vi "XY Graph Delete Plot.vi"(8 "Error In":errorcluster, 9 "Plot Index":i32, 11 "XYGraph Ref":T1) -> (0 "Error Out":errorcluster, 2 "Plot Name":string, 3 "XYGraph Ref":T1, 5 "Graph Caption (or Label)":string)   [LabVIEW 2019, in "XY Graph Add-Ons.lvlib"]
uses:
  XY Graph Add-Ons.lvlib
  XY Graph Refnum.ctl
  Plot Update Steps.ctl
  XY Graph Plot Properties.ctl
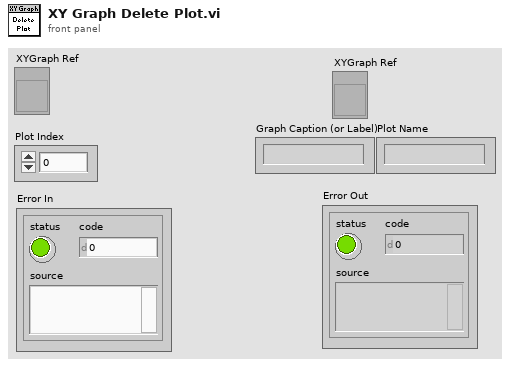
[diagram p1: front panel]
types:
  T1 = typedef "XY Graph Add-Ons.lvlib/XY Graph Refnum.ctl" = refnum<vi>
  T2 = typedef "Plot Update Steps.ctl" = enum16{"Update Plot Styles", "Update Annotation List", "Update Cursor List", "Update Plots", "Quit"}
  T3 = typedef "XY Graph Plot Properties.ctl" = cluster{"Plot Index":i32, "Plot.Bar Plot Style":u8, "Plot.DigitalLineStyle":u8, "Plot.TransitionLocation":u8, "Plot.Transition Type":u8, "Plot.Fill To":i16, "Plot.Fill/Pt. Color":u32, "Plot.Label Format":u8, "Plot.Line Style":u8, "Plot.Line Width":u8, "Plot.Plot Color":u32, "Plot.Plot Interpolation":u8, "Plot.Plot Name":string, "Plot.Point Style":u8, "Plot.Visible?":bool, "Plot.XScaleIdx":u32, "Plot.YScaleIdx":u32, "Plot.Anti-aliased":bool}
  T4 = typedef "LVAnnotationListTypeDef.ctl" = cluster{"Name":string, "Color":u32, "Style":u8, "Point Style":u8, "Name Visible":bool, "Allow Drag":bool, "Annotation Mode":u32, "Plot":i32, "Index":i32, "Position":cluster{"X":dbl, "Y":dbl}, "X Scale":u32, "Y Scale":u32, "Show Arrow":bool, "Lock Name":bool, "Plot Area":i32, "Label Offset":cluster{"X":dbl, "Y":dbl}}[]
  T5 = typedef "LVCursorListTypeDef.ctl" = cluster{"Name":string, "Color":u32, "Style":u8, "Point Style":u8, "Name Visible":bool, "Allow Drag":bool, "Cursor Mode":u32, "Plot":i32, "Index":i32, "Position":cluster{"X":dbl, "Y":dbl}, "X Scale":u32, "Y Scale":u32, "Watch Plots":i32[], "Watch All Plots":bool, "Plot Area":i32, "Label Offset":cluster{"X":dbl, "Y":dbl}}[]
  T6 = cluster{"Name":string, "Color":u32, "Style":u8, "Point Style":u8, "Name Visible":bool, "Allow Drag":bool, "Annotation Mode":u32, "Plot":i32, "Index":i32, "Position":cluster{"X":dbl, "Y":dbl}, "X Scale":u32, "Y Scale":u32, "Show Arrow":bool, "Lock Name":bool, "Plot Area":i32, "Label Offset":cluster{"X":dbl, "Y":dbl}}
  T7 = cluster{"Name":string, "Color":u32, "Style":u8, "Point Style":u8, "Name Visible":bool, "Allow Drag":bool, "Cursor Mode":u32, "Plot":i32, "Index":i32, "Position":cluster{"X":dbl, "Y":dbl}, "X Scale":u32, "Y Scale":u32, "Watch Plots":i32[], "Watch All Plots":bool, "Plot Area":i32, "Label Offset":cluster{"X":dbl, "Y":dbl}}
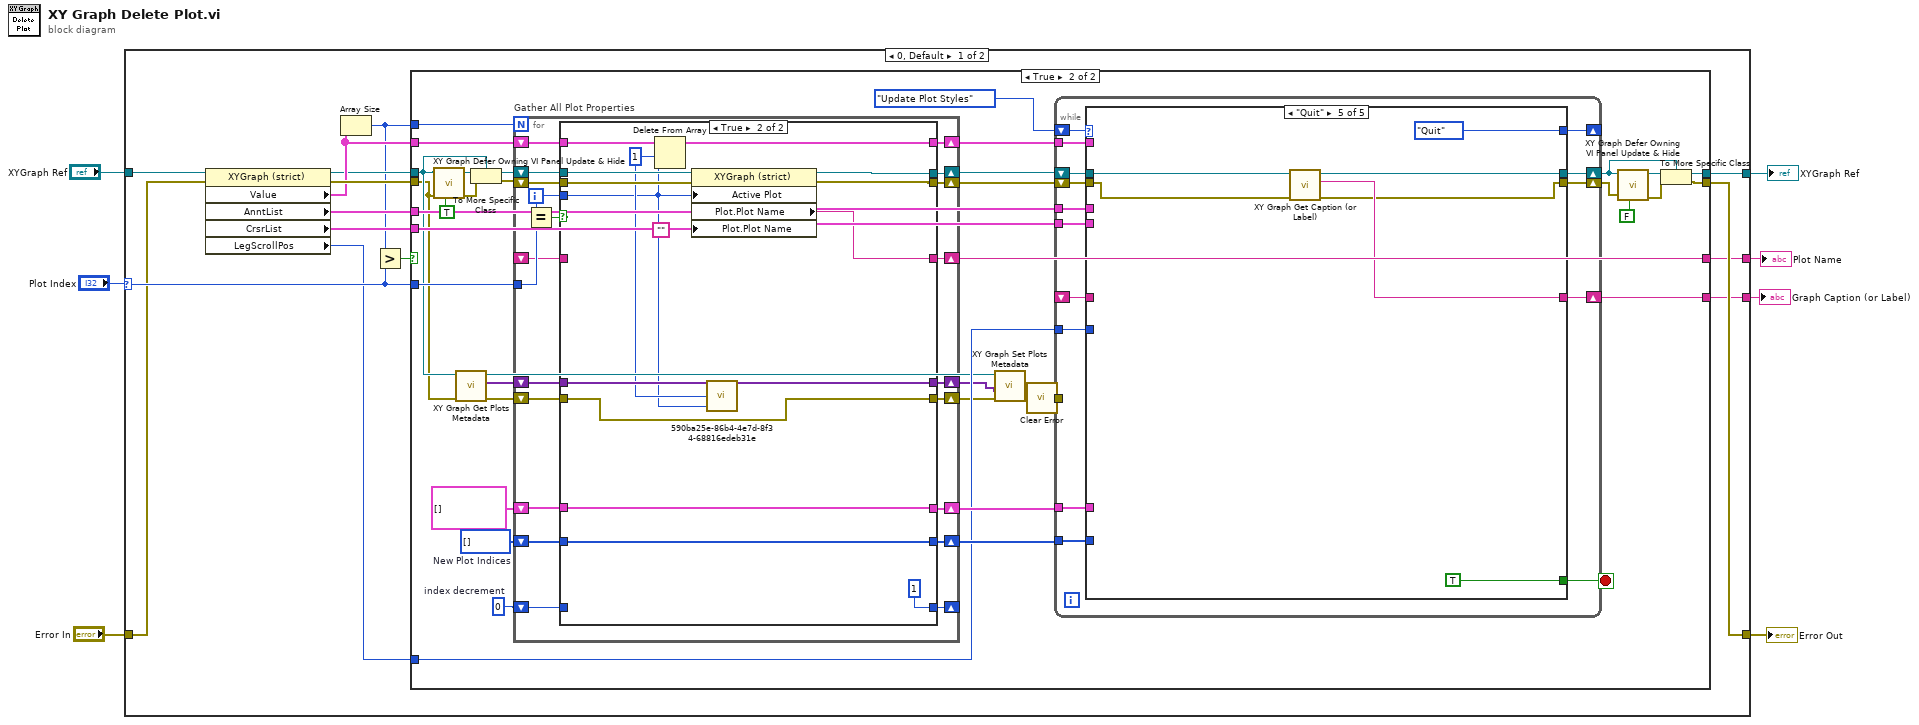
[diagram p0: block diagram]
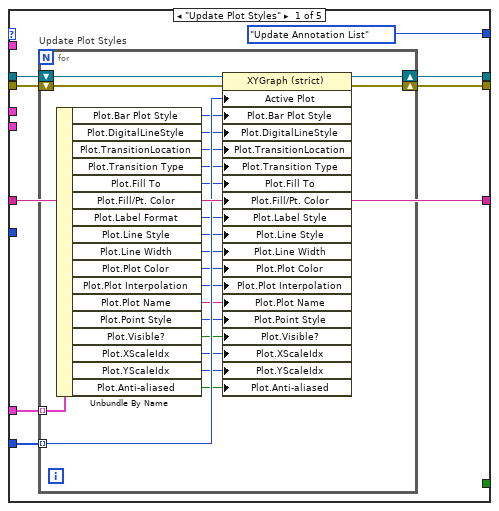
[diagram p3: hidden frame]
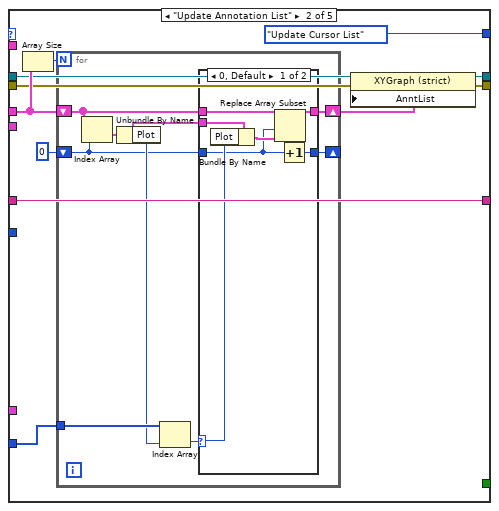
[diagram p4: hidden frame]
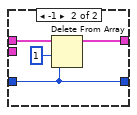
[diagram p5: hidden frame]
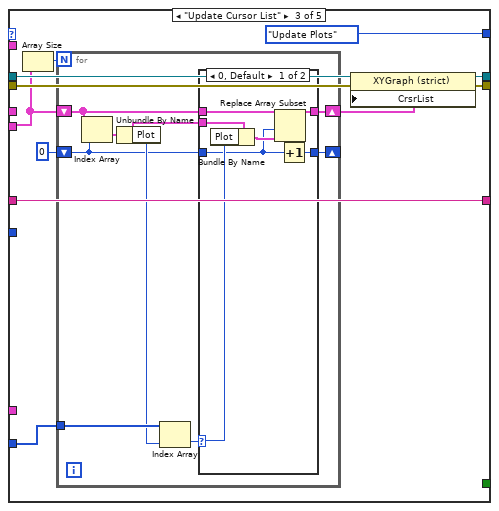
[diagram p6: hidden frame]
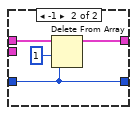
[diagram p7: hidden frame]
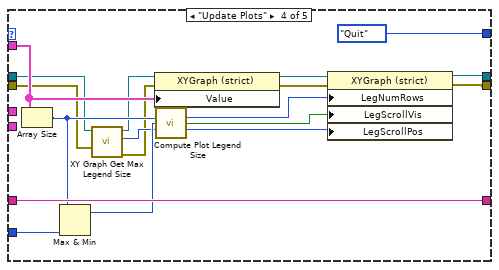
[diagram p8: hidden frame]
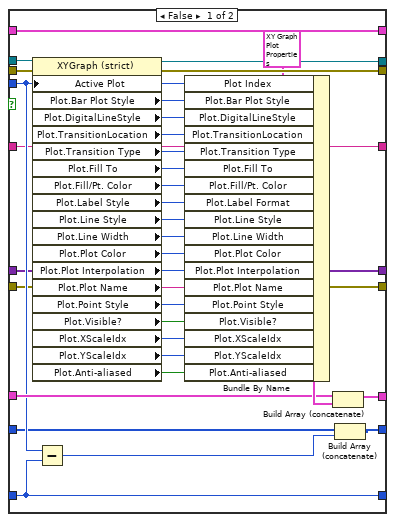
[diagram p9: hidden frame]
diagram:
  n1 = case shown="0, Default" "Plot Index" {
    selector: "Plot Index" -> [w13 _]
    tunnel: "XYGraph Ref" -> [w9 w266]
    tunnel: [w19 w266] -> w5
    tunnel: "Error In" -> [w8 w265]
    tunnel: [w18 w265] -> w3
    tunnel: [w15 _] -> w2
    tunnel: [w14 _] -> w1
    frame 0, Default {
      n2 = property class="XYGraph (strict)"(reference=w9, error in=w8) -> (reference out=w16:T1, error out=w22:errorcluster, "Value"=w21:cluster{"X Array":dbl[], "Y Array":dbl[]}[], "AnntList"=w20:T4, "CrsrList"=w17:T5, "LegScrollPos"=w10:u32)
      n3 = Array Size(array=w21) -> (size(s)=w12:i32)
      n4 = Greater?(x=w12, y=w13) -> (0:w11:bool)
      n5 = case shown="True" w11 {
        tunnel: w22 -> [w23 w32]
        tunnel: w21 -> [_ w61]
        tunnel: w20 -> [_ w55]
        tunnel: [w24 w37] -> w19
        tunnel: [w23 w34] -> w18
        tunnel: w17 -> [_ w53]
        tunnel: w16 -> [w24 w33]
        tunnel: [_ w52] -> w15
        tunnel: [_ w51] -> w14
        tunnel: w13 -> [_ w50]
        tunnel: w12 -> [_ w49]
        tunnel: w10 -> [_ w48]
        frame False {
        }
        frame True {
          w58 = i32[] []  # New Plot Indices
          w60 = 0  # index decrement
          n6 = call "XY Graph Defer Owning VI Panel Update & Hide.vi"("Defer Owning Panel Update"=TRUE, "error in (no error)"=w32, "XY Graph Refnum in"=w33) -> ("error out"=w39:errorcluster, "XY Graph Refnum out"=w41:refnum<vi>)  [unwired: 7 in]
          n7 = call "XY Graph Get Plots Metadata.vi"("Error In"=w32, "XYGraph Refnum"=w33) -> ("Error Out"=w31:errorcluster, "Plots Metadata"=w30:variant[], "XYGraph Refnum"=w26:T1)  [unwired: 6 in, 1 out]
          n8 = To More Specific Class(target class=w33, reference=w41, error in=w39) -> (specific class reference=w40:T1, error out=w38:errorcluster)
          n9 = for "Gather All Plot Properties" {
            N: w49 -> [_]
            tunnel: w50 -> [w212]
            shift-right: [w209] -> w54
            shift-left: w61 -> [w210]
            shift-right: [w204] -> w59
            shift-left: T3[] [] -> [w205]
            shift-right: [w206] -> w46
            shift-left: w38 -> [w207]
            shift-right: [w202] -> _
            shift-left: w60 -> [w203]
            shift-right: [w200] -> w57
            shift-left: w58 -> [w201]
            shift-right: [w208] -> w47
            shift-left: w40 -> [w214]
            shift-right: [w199] -> w51
            shift-left: _ -> [w198]
            shift-right: [w196] -> w29
            shift-left: w31 -> [w197]
            shift-right: [w194] -> w25
            shift-left: w30 -> [w195]
            i -> [w213]
            n10 = Equal?(x=w213, y=w212) -> (x = y?=w211:bool)
            n11 = case shown="True" w211 {
              tunnel: w214 -> [w248 w262]
              tunnel: w213 -> [w223 w251]
              tunnel: w210 -> [w247 w264]
              tunnel: [w247 w263] -> w209
              tunnel: [w246 w258] -> w208
              tunnel: w207 -> [w245 w257]
              tunnel: [w244 w256] -> w206
              tunnel: w205 -> [w225 w261]
              tunnel: [w224 w261] -> w204
              tunnel: w203 -> [w222 _]
              tunnel: [w222 1 ("index decrement")] -> w202
              tunnel: w201 -> [w221 w259]
              tunnel: [w219 w259] -> w200
              tunnel: [w218 w255] -> w199
              tunnel: w198 -> [w218 _]
              tunnel: w197 -> [w216 w249]
              tunnel: [w216 w249] -> w196
              tunnel: w195 -> [w215 w253]
              tunnel: [w215 w250] -> w194
              frame False {
                n12 = property class="XYGraph (strict)"(reference=w248, error in=w245, "Active Plot"=w223) -> (reference out=w246:T1, error out=w244:errorcluster, "Plot.Bar Plot Style"=w243:u8, "Plot.DigitalLineStyle"=w242:u8, "Plot.TransitionLocation"=w241:u8, "Plot.Transition Type"=w240:u8, "Plot.Fill To"=w239:i16, "Plot.Fill/Pt. Color"=w238:u32, "Plot.Label Style"=w237:u8, "Plot.Line Style"=w236:u8, "Plot.Line Width"=w235:u8, "Plot.Plot Color"=w234:u32, "Plot.Plot Interpolation"=w233:u8, "Plot.Plot Name"=w232:string, "Plot.Point Style"=w231:u8, "Plot.Visible?"=w230:bool, "Plot.XScaleIdx"=w229:u32, "Plot.YScaleIdx"=w228:u32, "Plot.Anti-aliased"=w217:bool)
                n13 = Subtract(x=w223, y=w222) -> (x-y=w220:i32)
                n14 = Bundle By Name(cluster=T3 {"Plot Index"=0, "Plot.Bar Plot Style"=0, "Plot.DigitalLineStyle"=0, "Plot.TransitionLocation"=0, "Plot.Transition Type"=0, "Plot.Fill To"=0, "Plot.Fill/Pt. Color"=0, "Plot.Label Format"=0, "Plot.Line Style"=0, "Plot.Line Width"=0, "Plot.Plot Color"=0, "Plot.Plot Interpolation"=0, "Plot.Plot Name"="", "Plot.Point Style"=0, "Plot.Visible?"=FALSE, "Plot.XScaleIdx"=0, "Plot.YScaleIdx"=0, "Plot.Anti-aliased"=FALSE}, "Plot Index"=w223, "Plot.Bar Plot Style"=w243, "Plot.DigitalLineStyle"=w242, "Plot.TransitionLocation"=w241, "Plot.Transition Type"=w240, "Plot.Fill To"=w239, "Plot.Fill/Pt. Color"=w238, "Plot.Label Format"=w237, "Plot.Line Style"=w236, "Plot.Line Width"=w235, "Plot.Plot Color"=w234, "Plot.Plot Interpolation"=w233, "Plot.Plot Name"=w232, "Plot.Point Style"=w231, "Plot.Visible?"=w230, "Plot.XScaleIdx"=w229, "Plot.YScaleIdx"=w228, "Plot.Anti-aliased"=w217) -> (w226:T3)
                n15 = Build Array (concatenate)(w225, w226) -> (w224:T3[])
                n16 = Build Array (concatenate)(w221, w220) -> (w219:i32[])
              }
              frame True {
                w252 = 1 ("length")
                n17 = Delete From Array(array=w264, length=w252, index=w251) -> (array with subset deleted=w263:cluster{"X Array":dbl[], "Y Array":dbl[]}[])  [unwired: 1 out]
                n18 = property class="XYGraph (strict)"(reference=w262, error in=w257, "Active Plot"=w251, "Plot.Plot Name"="") -> (reference out=w258:T1, error out=w256:errorcluster, "Plot.Plot Name"=w255:string)
                n19 = call "590ba25e-86b4-4e7d-8f34-68816edeb31e.vi"("index (last elem)"=w251, "length (1)"=w252, "Array"=w253) -> ("array w/ subset deleted"=w250:variant[])  [unwired: 1 out]
              }
            }
          }
          n20 = call "XY Graph Set Plots Metadata.vi"("error in (no error)"=w29, "Plots Metadata"=w25, "XY Graph Refnum"=w26) -> ("error out"=w28:errorcluster)  [unwired: 7 in, 1 out]
          n21 = call "Clear Error.vi"("Error In"=w28) -> ("no Error Out"=w27:errorcluster)  [unwired: 8 in]
          n22 = while {
            tunnel: w59 -> [w77]
            tunnel: w57 -> [w74]
            shift-right: [w71] -> _
            shift-left: Plot_Update_Steps."Update Plot Styles" -> [w73]
            shift-right: [w63] -> w43
            shift-left: w46 -> [w75]
            tunnel: w55 -> [w70]
            tunnel: w54 -> [w69]
            tunnel: w53 -> [w68]
            shift-right: [w64] -> w36
            shift-left: w47 -> [w76]
            shift-right: [w67] -> w52
            shift-left: _ -> [w66]
            tunnel: w48 -> [w65]
            tunnel: w27 -> [_]
            stop <- w72 stop-if-true
            n23 = case shown="\"Quit\"" w73 {
              tunnel: w77 -> [w85 _ _ _ _]
              tunnel: w76 -> [w84 w114 w145 w171 w192]
              tunnel: w75 -> [w83 w112 w143 w169 w188]
              tunnel: [w82 w111 w142 w182 w187] -> w63
              tunnel: [w81 w113 w144 w183 w189] -> w64
              tunnel: w74 -> [w80 w118 w148 _ _]
              tunnel: [_ _ _ _ TRUE] -> w72
              tunnel: [Plot_Update_Steps."Update Annotation List" Plot_Update_Steps."Update Cursor List" Plot_Update_Steps."Update Plots" Plot_Update_Steps."Quit" Plot_Update_Steps."Quit"] -> w71
              tunnel: w70 -> [_ w117 _ _ _]
              tunnel: w69 -> [_ _ _ w185 _]
              tunnel: w68 -> [_ _ w140 _ _]
              tunnel: [w78 w109 w139 w180 w190] -> w67
              tunnel: w66 -> [w78 w109 w139 w180 _]
              tunnel: w65 -> [_ _ _ w178 _]
              frame "Update Plot Styles" {
                n24 = for "Update Plot Styles" {
                  tunnel: w85 -> [w108] mode=indexing
                  shift-right: [w104] -> w82
                  shift-left: w83 -> [w105]
                  tunnel: w80 -> [w103] mode=indexing
                  shift-right: [w106] -> w81
                  shift-left: w84 -> [w107]
                  n25 = Unbundle By Name(w108) -> ("Plot.Bar Plot Style"=w102:u8, "Plot.DigitalLineStyle"=w101:u8, "Plot.TransitionLocation"=w100:u8, "Plot.Transition Type"=w99:u8, "Plot.Fill To"=w98:i16, "Plot.Fill/Pt. Color"=w97:u32, "Plot.Label Format"=w96:u8, "Plot.Line Style"=w95:u8, "Plot.Line Width"=w94:u8, "Plot.Plot Color"=w93:u32, "Plot.Plot Interpolation"=w92:u8, "Plot.Plot Name"=w91:string, "Plot.Point Style"=w90:u8, "Plot.Visible?"=w89:bool, "Plot.XScaleIdx"=w88:u32, "Plot.YScaleIdx"=w87:u32, "Plot.Anti-aliased"=w86:bool)
                  n26 = property class="XYGraph (strict)"(reference=w107, error in=w105, "Active Plot"=w103, "Plot.Bar Plot Style"=w102, "Plot.DigitalLineStyle"=w101, "Plot.TransitionLocation"=w100, "Plot.Transition Type"=w99, "Plot.Fill To"=w98, "Plot.Fill/Pt. Color"=w97, "Plot.Label Style"=w96, "Plot.Line Style"=w95, "Plot.Line Width"=w94, "Plot.Plot Color"=w93, "Plot.Plot Interpolation"=w92, "Plot.Plot Name"=w91, "Plot.Point Style"=w90, "Plot.Visible?"=w89, "Plot.XScaleIdx"=w88, "Plot.YScaleIdx"=w87, "Plot.Anti-aliased"=w86) -> (reference out=w106:T1, error out=w104:errorcluster)
                }
              }
              frame "Update Annotation List" {
                n27 = Array Size(array=w117) -> (size(s)=w116:i32)
                n28 = for {
                  N: w116 -> [_]
                  tunnel: w118 -> [w127]
                  shift-right: [w121] -> w110
                  shift-left: w117 -> [w123]
                  shift-right: [w120] -> _
                  shift-left: 0 -> [w122]
                  n29 = Index Array(array=w123, index=w122) -> (element=w125:T6)
                  n30 = Unbundle By Name(w125) -> ("Plot"=w126:i32)
                  n31 = Index Array(array=w127, index=w126) -> (element=w124:i32)
                  n32 = case shown="0, Default" w124 {
                    selector: w124 -> [w133 _]
                    tunnel: w125 -> [w134 _]
                    tunnel: w123 -> [w131 w138]
                    tunnel: w122 -> [w129 w135]
                    tunnel: [w128 w136] -> w121
                    tunnel: [w132 w135] -> w120
                    frame 0, Default {
                      n33 = Bundle By Name(cluster=w134, "Plot"=w133) -> (w130:T6)
                      n34 = Replace Array Subset(array=w131, new element=w130, index=w129) -> (w128:T4)
                      n35 = Increment(x=w129) -> (x+1=w132:i32)
                    }
                    frame -1 {
                      n36 = Delete From Array(array=w138, length=1, index=w135) -> (array with subset deleted=w136:T4)  [unwired: 1 out]
                    }
                  }
                }
                n37 = property class="XYGraph (strict)"(reference=w114, error in=w112, "AnntList"=w110) -> (reference out=w113:T1, error out=w111:errorcluster)
              }
              frame "Update Cursor List" {
                n38 = Array Size(array=w140) -> (size(s)=w147:i32)
                n39 = for {
                  N: w147 -> [_]
                  tunnel: w148 -> [w157]
                  shift-right: [w151] -> w141
                  shift-left: w140 -> [w153]
                  shift-right: [w150] -> _
                  shift-left: 0 -> [w152]
                  n40 = Index Array(array=w153, index=w152) -> (element=w155:T7)
                  n41 = Unbundle By Name(w155) -> ("Plot"=w156:i32)
                  n42 = Index Array(array=w157, index=w156) -> (element=w154:i32)
                  n43 = case shown="0, Default" w154 {
                    selector: w154 -> [w163 _]
                    tunnel: w155 -> [w164 _]
                    tunnel: w153 -> [w161 w168]
                    tunnel: w152 -> [w159 w165]
                    tunnel: [w158 w166] -> w151
                    tunnel: [w162 w165] -> w150
                    frame 0, Default {
                      n44 = Bundle By Name(cluster=w164, "Plot"=w163) -> (w160:T7)
                      n45 = Replace Array Subset(array=w161, new element=w160, index=w159) -> (w158:T5)
                      n46 = Increment(x=w159) -> (x+1=w162:i32)
                    }
                    frame -1 {
                      n47 = Delete From Array(array=w168, length=1, index=w165) -> (array with subset deleted=w166:T5)  [unwired: 1 out]
                    }
                  }
                }
                n48 = property class="XYGraph (strict)"(reference=w145, error in=w143, "CrsrList"=w141) -> (reference out=w144:T1, error out=w142:errorcluster)
              }
              frame "Update Plots" {
                n49 = Array Size(array=w185) -> (size(s)=w177:i32)
                n50 = Max & Min(x=w177, y=w178) -> (max(x,y)=w179:u32)  [unwired: 1 out]
                n51 = call "XY Graph Get Max Legend Size.vi"("Error In"=w169, "XYGraph Refnum"=w171) -> ("Error Out"=w170:errorcluster, "Max Legend Size"=w173:i32, "XYGraph Refnum"=w172:T1)  [unwired: 6 in, 1 out]
                n52 = property class="XYGraph (strict)"(reference=w172, error in=w170, "Value"=w185) -> (reference out=w184:T1, error out=w181:errorcluster)
                n53 = call "Compute Plot Legend Size.vi"("# Plots"=w177, "Current Plot (Last)"=w179, "Max Legend Size"=w173) -> ("LegNumRows"=w176:u32, "LegScrollVis"=w175:bool, "LegScrollPos"=w174:u32)  [unwired: 10 in]
                n54 = property class="XYGraph (strict)"(reference=w184, error in=w181, "LegNumRows"=w176, "LegScrollVis"=w175, "LegScrollPos"=w174) -> (reference out=w183:T1, error out=w182:errorcluster)
              }
              frame "Quit" {
                n55 = call "XY Graph Get Caption (or Label).vi"("error in (no error)"=w188, "XYGraph in"=w192) -> ("error out"=w187:errorcluster, "Caption (or Label) Text"=w190:string, "XYGraph out"=w189:T1)  [unwired: 7 in]
              }
            }
          }
          n56 = call "XY Graph Defer Owning VI Panel Update & Hide.vi"("Defer Owning Panel Update"=FALSE, "error in (no error)"=w43, "XY Graph Refnum in"=w36) -> ("error out"=w35:errorcluster, "XY Graph Refnum out"=w44:refnum<vi>)  [unwired: 7 in]
          n57 = To More Specific Class(target class=w36, reference=w44, error in=w35) -> (specific class reference=w37:T1, error out=w34:errorcluster)
        }
      }
    }
    frame ..-1 {
    }
  }
  "XYGraph Ref" <- w5
  "Error Out" <- w3
  "Graph Caption (or Label)" <- w2
  "Plot Name" <- w1
